vi "ep_Calculate t0.vi"(7 "dt":dbl, 8 "freq":dbl, 9 "y2":dbl, 10 "y1":dbl, 11 "t1":i32) -> (3 "t0":dbl)   [LabVIEW 2012, in "NI_EP_Resample_Host.lvlib"]
uses:
  <vilib>/addons/Electrical Power/PQ/Resampling/NI_EP_Resample_Host.lvlib
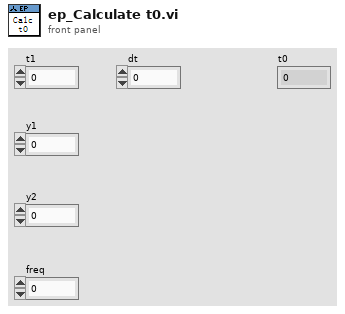
[diagram p1: front panel]
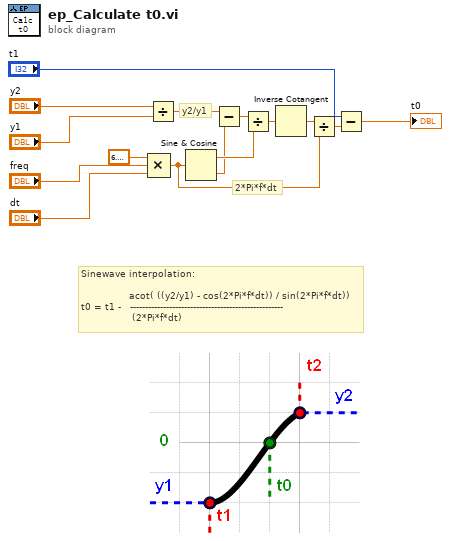
[diagram p0: block diagram]
diagram:
  # "y2/y1"
  # "2*Pi*f*dt"
  # "Sinewave interpolation:\n\n                acot( ((y2/y1) - cos(2*Pi*f*dt)) / sin(2*Pi*f*dt))\nt0 = t1 -   ---------------------------------------------------\n                 (2*Pi*f*dt)"
  n1 = Divide(x="y2", y="y1") -> (x/y=w1:dbl)
  n2 = Compound Arithmetic op=MULTIPLY(sgl 6.2831855, "freq", "dt") -> (w7:dbl)
  n3 = Sine & Cosine(0:w7) -> (1:w9:dbl, 2:w8:dbl)
  n4 = Subtract(x=w1, y=w8) -> (x-y=w2:dbl)
  n5 = Divide(x=w2, y=w9) -> (x/y=w3:dbl)
  n6 = Inverse Cotangent(1:w3) -> (0:w4:dbl)
  n7 = Divide(x=w4, y=w7) -> (x/y=w5:dbl)
  n8 = Subtract(x="t1", y=w5) -> (x-y=→"t0":dbl)
